vi "Load Manager Subpanel.vi"(8 "error in (no error)":errorcluster, 9 "Calling VI":refnum<vi>, 10 "Subpanel Type":T1, 11 "CIF_UI in":refnum<class "CIF_Manager_UI.lvclass">) -> (0 "error out":errorcluster, 2 "VI Reference":refnum<vi>, 3 "CIF_UI out":refnum<class "CIF_Manager_UI.lvclass">)   [LabVIEW 2021, in "CIF_Manager_UI.lvclass"]
uses:
  CIF_Manager_UI.lvclass
  C:/Program Files/National Instruments/LabVIEW 2021/vi.lib/CIF Foundation/CIF Core/CIFUI/CIF_UI.lvclass
  Typedef/Manager Subpanel Type.ctl
  <vilib>/CIF Foundation/CIF Core/CIFUI/CIF_UI.lvclass/CIF_UI.ctl
  CIF_Manager_UI.lvclass/CIF_Manager_UI.ctl
  Typedef/Class Data for Manager SubPanel.ctl
  <vilib>/gRPC/LabVIEW gRPC Library/Shared/grpcId.ctl
  <vilib>/CIF Foundation/CIF Core/CIFUI/Typedef/Core UI References.ctl
  <vilib>/CIF Foundation/CIF Core/CIFUI/Typedef/SubPanel Events.ctl
  <vilib>/CIF Foundation/CIF Core/CIFUI/Typedef/New Connection Event Data.ctl
  <vilib>/CIF Foundation/CIF Core/CIFUI/Typedef/New Connection Plugin Event Data.ctl
  Typedef/Core Manager UI References.ctl
  <vilib>/CIF Foundation/CIF Core/CIFUI/Typedef/Subpanel Data.ctl
  <vilib>/CIF Foundation/CIF Core/CIFUI/Typedef/Plugin Subpanel Events.ctl
  <vilib>/CIF Foundation/CIF Core/CIFCore/Common/Typedef/Errors.ctl
  <vilib>/CIF Foundation/CIF Utilities/Errors/Append Error Location.vi
  <vilib>/Utility/LVLibp/NI_PackedLibraryUtility.lvlib
  78e05929-4a52-4a7a-a51a-d61806b701c4.vi
  <vilib>/CIF Foundation/CIF Core/CIFCore/Common/CIFCoreCommon.lvlib
  <vilib>/CIF Foundation/CIF Core/CIFUtilities/CIFConfigurationFile/typedef/Location Type.ctl
  <vilib>/CIF Foundation/CIF Core/CIFUtilities/CIFConfigurationFile/CIF Configuration File.lvlib
  <vilib>/CIF Foundation/CIF Core/CIFUI/CIF_UI.lvclass
  <vilib>/gRPC/LabVIEW gRPC Library/grpc-lvsupport-release.lvlib
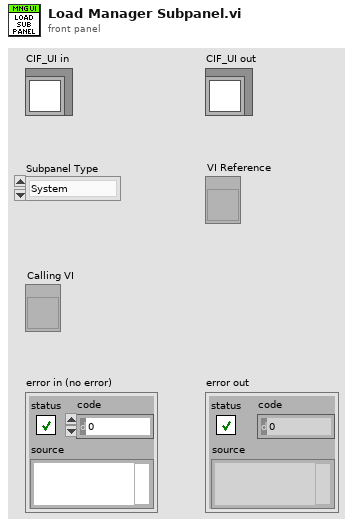
[diagram p1: front panel]
types:
  T1 = typedef "CIF_Manager_UI.lvclass/Manager Subpanel Type.ctl" = enum16{"System", "Errors", "Channel", "Plugin"}
  T2 = typedef "CIF_Manager_UI.lvclass/Class Data for Manager SubPanel.ctl" = cluster{"Class Data for SubPanel":cluster{"IP Address":string, "Manager gRPC ID":T3, "Server Certificate File (.crt)":path, "Connected":bool, "Manager Connection":bool, "Core UI References":T4, "Subpanel Events":T5}, "Manager UI References":T6}
  T3 = typedef "grpc-lvsupport-release.lvlib/grpcId.ctl" = u64
  T4 = typedef "CIF_UI.lvclass/Core UI References.ctl" = cluster{"Plugin Status":refnum<vi>, "Plugin Status Valid":bool, "Connection":refnum<vi>, "Connection Valid":bool, "Exit":refnum<vi>, "Exit Valid":bool, "Run Listen":refnum<vi>, "Run Listen Valid":bool, "Clear Local Error":refnum<vi>, "Clear Local Error Valid":bool, "Local Error":refnum<vi>, "Local Error Valid":bool}
  T5 = typedef "CIF_UI.lvclass/SubPanel Events.ctl" = cluster{"Clear Local Error":refnum<user-event>, "Shutdown":refnum<user-event>, "gRPC Connection":refnum<user-event>, "Plugin Connection":refnum<user-event>}
  T6 = typedef "CIF_Manager_UI.lvclass/Core Manager UI References.ctl" = cluster{"Discovered Plugins":refnum<vi>, "Discovered Plugins Valid":bool, "Loaded Plugins":refnum<vi>, "Loaded Plugins Valid":bool, "Publisher Channels":refnum<vi>, "Publisher Channels Valid":bool, "Subscriber Channels":refnum<vi>, "Subscriber Channels Valid":bool, "Channel Connection":refnum<vi>, "Channel Connection Valid":bool, "New Plugin Load":refnum<vi>, "New Plugin Load Valid":bool, "Errors":refnum<vi>, "Errors Valid":bool, "Plugin to Abort":refnum<vi>, "Plugin to Abort Valid":bool, "CIF Manager Tab":refnum<vi>, "Manger Tab Valid":bool, "System Errors":refnum<vi>, "System Errors Valid":bool, "Plugin Selection":refnum<vi>, "Plugin Selection Valid":bool}
  T7 = typedef "CIF_UI.lvclass/Subpanel Data.ctl" = cluster{"VI Reference":refnum<vi>, "Plugin Subpanel Events":T8}
  T8 = typedef "CIF_UI.lvclass/Plugin Subpanel Events.ctl" = cluster{"Plugin Shutdown":refnum<user-event>}
  T9 = typedef "CIFCoreCommon.lvlib/Errors.ctl" = enum16{"Invalid Clock ID", "Long Sleep", "gRPC Server Not Found", "Config Parse", "Timestamp Wrap", "Delayed Execution", "Duplicate Channel", "Missing Channel", "Incorrect Type", "Flatten Error", "Unflatten Data", "Unique Name", "Plugin Not Found", "Plugin Type Not Found", "Plugin Version Not Found", "Manager Not Found", "Numerical Issue", "Time Jump", "Clock ID Match", "Channel Length", "Plugin Connection", "gRPC Server Connection", "PPL Name Match", "Build", "Config Log Parse", "Plugin Load", "UI Subpanel Load", "Python Name", "Invalid Name", "Unable to Change Ch Buffer", "Failed Kill", "Failed SysExec", "Function Not Implemented", "Load Timeout"}
  T10 = typedef "CIF Configuration File.lvlib/Location Type.ctl" = enum16{"Config File", "Manager", "Protos", "Plugins", "UI Plugins", "Logs", "Orchestrations", "Loaders"}
  T11 = typedef "CIF_UI.lvclass/Class Data for SubPanel.ctl" = cluster{"IP Address":string, "Manager gRPC ID":T3, "Server Certificate File (.crt)":path, "Connected":bool, "Manager Connection":bool, "Core UI References":T4, "Subpanel Events":T5}
  T12 = typedef "CIF_Manager_UI.lvclass/Manager Subpanel Map.ctl" = map{T1, T7}
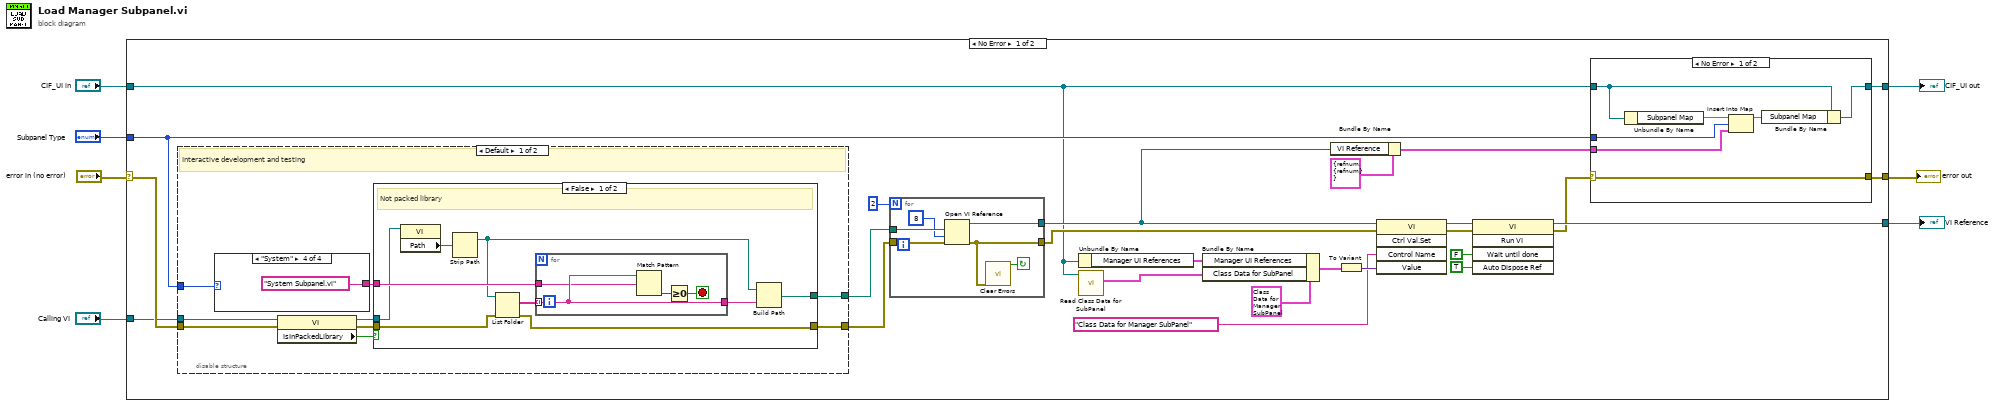
[diagram p0: block diagram]
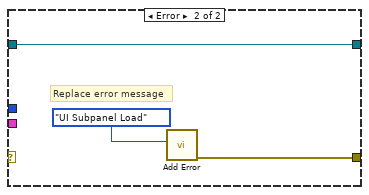
[diagram p2: hidden frame]
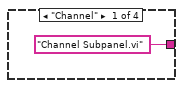
[diagram p3: hidden frame]
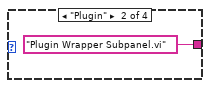
[diagram p4: hidden frame]
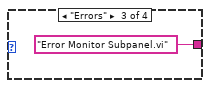
[diagram p5: hidden frame]
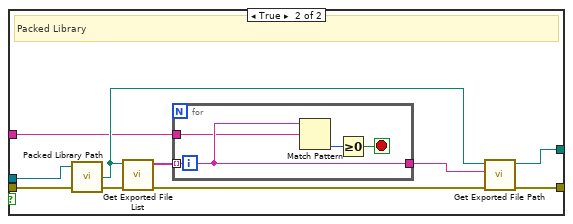
[diagram p6: hidden frame]
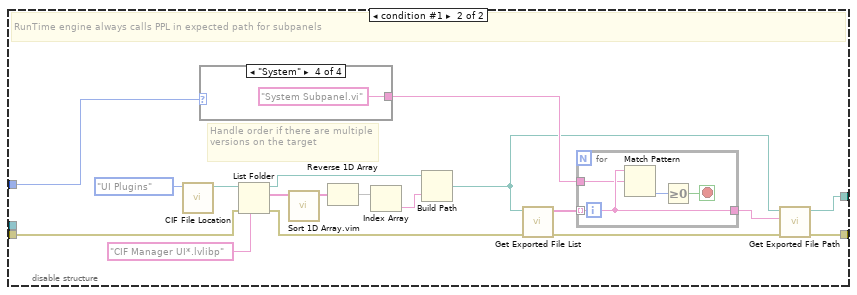
[diagram p7: hidden frame]
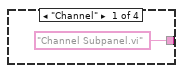
[diagram p8: hidden frame]
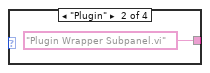
[diagram p9: hidden frame]
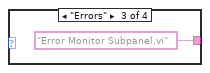
[diagram p10: hidden frame]
diagram:
  n1 = case shown="No Error" "error in (no error)" {
    selector: "error in (no error)" -> [w20 w116]
    tunnel: [w15 w116] -> w6
    tunnel: [w23 w115] -> w4
    tunnel: "CIF_UI in" -> [w12 w115]
    tunnel: "Subpanel Type" -> [w17 _]
    tunnel: [w22 _] -> w2
    tunnel: "Calling VI" -> [w16 _]
    frame No Error {
      n2 = disable-structure shown="Default" {
        disable-tunnel: w20 -> [w48 w87]
        disable-tunnel: [w47 w100] -> w19
        disable-tunnel: [w46 w99] -> w18
        disable-tunnel: w17 -> [w44 w83]
        disable-tunnel: w16 -> [w43 _]
        frame condition #0 (active) {
          # "Interactive development and testing"
          n3 = case shown="\"System\"" w44 {
            tunnel: ["Channel Subpanel.vi" ("regular expression") "Plugin Wrapper Subpanel.vi" ("regular expression") "Error Monitor Subpanel.vi" ("regular expression") "System Subpanel.vi" ("regular expression")] -> w45
            frame "Channel" {
            }
            frame "Plugin" {
            }
            frame "Errors" {
            }
            frame "System" {
            }
          }
          n4 = property class="VI"(reference=w43, error in=w48) -> (reference out=w50:refnum<vi>, error out=w51:errorcluster, "IsInPackedLibrary"=w49:bool)
          n5 = case shown="False" w49 {
            tunnel: w50 -> [w58 w78]
            tunnel: w51 -> [w62 w77]
            tunnel: [w56 w69] -> w46
            tunnel: [w61 w71] -> w47
            tunnel: w45 -> [w63 w70]
            frame False {
              # "Not packed library"
              n6 = property class="VI"(reference=w58) -> ("Path"=w59:path)  [unwired: 1 in, 2 out]
              n7 = Strip Path(path=w59) -> (stripped path=w60:path)  [unwired: 1 out]
              n8 = List Folder(path=w60, error in=w62) -> (filenames=w64:string[], error out=w61:errorcluster)  [unwired: 2 in, 2 out]
              n9 = for {
                tunnel: w64 -> [w66] mode=indexing
                tunnel: [w66] -> w57
                tunnel: w63 -> [w65]
                stop <- w67 stop-if-true
                n10 = Match Pattern(string=w66, regular expression=w65) -> (offset past match=w68:i32)  [unwired: 1 in, 3 out]
                n11 = Greater Or Equal To 0?(x=w68) -> (x >= 0?=w67:bool)
              }
              n12 = Build Path(base path=w60, name or relative path=w57) -> (appended path=w56:path)
            }
            frame True {
              # "Packed Library"
              n13 = call <vilib>:"Packed Library Path.vi"("error in (no error)"=w77, "vi reference"=w78) -> ("error out"=w72:errorcluster, "packed library path"=w73:path)  [unwired: 1 in, 1 out]
              n14 = call <vilib>:"Get Exported File List.vi"("error in (no error)"=w72, "packed library path"=w73) -> ("error out"=w75:errorcluster, "qualified names"=w74:string[])  [unwired: 7 in, 1 out]
              n15 = for {
                tunnel: w74 -> [w80] mode=indexing
                tunnel: [w80] -> w76
                tunnel: w70 -> [w79]
                stop <- w81 stop-if-true
                n16 = Match Pattern(string=w80, regular expression=w79) -> (offset past match=w82:i32)  [unwired: 1 in, 3 out]
                n17 = Greater Or Equal To 0?(x=w82) -> (x >= 0?=w81:bool)
              }
              n18 = call <vilib>:"Get Exported File Path.vi"("error in (no error)"=w75, "qualified name"=w76, "packed library path"=w73) -> ("error out"=w71:errorcluster, "path"=w69:path)  [unwired: 7 in]
            }
          }
        }
        frame condition #1 {
          # "Handle order if there are multiple versions on the target"
          # "RunTime engine always calls PPL in expected path for subpanels"
          n19 = call <vilib>:"CIF File Location.vi"("LocationType"=Location_Type."UI Plugins") -> ("Location"=w84:path)  [unwired: 10 in]
          n20 = case shown="\"System\"" w83 {
            tunnel: ["Channel Subpanel.vi" ("regular expression") "Plugin Wrapper Subpanel.vi" ("regular expression") "Error Monitor Subpanel.vi" ("regular expression") "System Subpanel.vi" ("regular expression")] -> w98
            frame "Channel" {
            }
            frame "Plugin" {
            }
            frame "Errors" {
            }
            frame "System" {
            }
          }
          n21 = List Folder(path=w84, pattern="CIF Manager UI*.lvlibp", error in=w87) -> (path out=w93:path, filenames=w90:string[], error out=w86:errorcluster)  [unwired: 1 in, 1 out]
          n22 = call "Sort 1D Array.vim"("unsorted array"=w90) -> ("sorted array"=w91:string[])  [unwired: 10 in]
          n23 = Reverse 1D Array(array=w91) -> (reversed array=w92:string[])
          n24 = Index Array(array=w92) -> (element=w94:string)  [unwired: 1 in]
          n25 = Build Path(base path=w93, name or relative path=w94) -> (appended path=w88:path)
          n26 = call <vilib>:"Get Exported File List.vi"("error in (no error)"=w86, "packed library path"=w88) -> ("error out"=w96:errorcluster, "qualified names"=w95:string[])  [unwired: 7 in, 1 out]
          n27 = for {
            tunnel: w95 -> [w102] mode=indexing
            tunnel: [w102] -> w97
            tunnel: w98 -> [w101]
            stop <- w103 stop-if-true
            n28 = Match Pattern(string=w102, regular expression=w101) -> (offset past match=w104:i32)  [unwired: 1 in, 3 out]
            n29 = Greater Or Equal To 0?(x=w104) -> (x >= 0?=w103:bool)
          }
          n30 = call <vilib>:"Get Exported File Path.vi"("error in (no error)"=w96, "qualified name"=w97, "packed library path"=w88) -> ("error out"=w100:errorcluster, "path"=w99:path)  [unwired: 7 in]
        }
      }
      n31 = for {
        N: 2 -> [_]
        tunnel: w18 -> [w114]
        tunnel: [w113] -> w21
        tunnel: [w112] -> w29
        tunnel: w19 -> [w110]
        stop <- w111 continue-if-true
        n32 = Open VI Reference(vi path=w114, options=8, error in (no error)=w110) -> (vi reference=w113:refnum<vi>, error out=w112:errorcluster)  [unwired: 3 in]
        n33 = call <vilib>:"Clear Errors.vi"("error in (no error)"=w112) -> ("specific error cleared?"=w111:bool)  [unwired: 5 in, 1 out]
      }
      n34 = Unbundle By Name(w12) -> ("Manager UI References"=w10:T6)
      n35 = call <vilib>:"Read Class Data for SubPanel.vi"("CIF_UI in"=w12) -> ("Class Data for SubPanel"=w9:T11)  [unwired: 8 in, 2 out]
      n36 = Bundle By Name(cluster=T2 {"Class Data for SubPanel"={"IP Address"="", "Manager gRPC ID"=0, "Server Certificate File (.crt)"=path "", "Connected"=FALSE, "Manager Connection"=FALSE, "Core UI References"={"Plugin Status"=refnum, "Plugin Status Valid"=FALSE, "Connection"=refnum, "Connection Valid"=FALSE, "Exit"=refnum, "Exit Valid"=FALSE, "Run Listen"=refnum, "Run Listen Valid"=FALSE, "Clear Local Error"=refnum, "Clear Local Error Valid"=FALSE, "Local Error"=refnum, "Local Error Valid"=FALSE}, "Subpanel Events"={"Clear Local Error"=refnum, "Shutdown"=refnum, "gRPC Connection"=refnum, "Plugin Connection"=refnum}}, "Manager UI References"={"Discovered Plugins"=refnum, "Discovered Plugins Valid"=FALSE, "Loaded Plugins"=refnum, "Loaded Plugins Valid"=FALSE, "Publisher Channels"=refnum, "Publisher Channels Valid"=FALSE, "Subscriber Channels"=refnum, "Subscriber Channels Valid"=FALSE, "Channel Connection"=refnum, "Channel Connection Valid"=FALSE, "New Plugin Load"=refnum, "New Plugin Load Valid"=FALSE, "Errors"=refnum, "Errors Valid"=FALSE, "Plugin to Abort"=refnum, "Plugin to Abort Valid"=FALSE, "CIF Manager Tab"=refnum, "Manger Tab Valid"=FALSE, "System Errors"=refnum, "System Errors Valid"=FALSE, "Plugin Selection"=refnum, "Plugin Selection Valid"=FALSE}} ("Class Data for Manager SubPanel"), "Manager UI References"=w10, "Class Data for SubPanel"=w9) -> (w8:T2)
      n37 = Bundle By Name(cluster=T7 {"VI Reference"=refnum, "Plugin Subpanel Events"={"Plugin Shutdown"=refnum}} ("SubPanel Data"), "VI Reference"=w21) -> (w24:T7)
      n38 = To Variant(anything=w8) -> (Variant=w25:variant)
      n39 = invoke class="VI" method="Ctrl Val.Set"(reference=w21, error in=w29, "Control Name"="Class Data for Manager SubPanel", "Value"=w25) -> (reference out=w30:refnum<vi>, error out=w31:errorcluster)  [unwired: 1 in, 3 out]
      n40 = invoke class="VI" method="Run VI"(reference=w30, error in=w31, "Wait until done"=FALSE ("Wait Until Done"), "Auto Dispose Ref"=TRUE ("Auto Dispose Reference")) -> (reference out=w22:refnum<vi>, error out=w13:errorcluster)  [unwired: 1 in, 3 out]
      n41 = case shown="No Error" w13 {
        selector: w13 -> [w33 _]
        tunnel: w24 -> [w38 _]
        tunnel: [w36 w42] -> w23
        tunnel: w17 -> [w35 _]
        tunnel: [w33 w41] -> w15
        tunnel: w12 -> [w34 w42]
        frame No Error {
          n42 = Unbundle By Name(w34) -> ("Subpanel Map"=w39:T12)
          n43 = Insert Into Map(map in=w39, key=w35, value=w38) -> (map out=w37:T12)  [unwired: 2 out]
          n44 = Bundle By Name(cluster=w34, "Subpanel Map"=w37) -> (w36:refnum<class "CIF_Manager_UI.lvclass">)
        }
        frame Error {
          # "Replace error message"
          n45 = call <vilib>:"Add Error.vi"("Error"=Errors."UI Subpanel Load") -> ("error out"=w41:errorcluster)  [unwired: 10 in]
        }
      }
    }
    frame Error {
    }
  }
  "error out" <- w6
  "CIF_UI out" <- w4
  "VI Reference" <- w2
